vi "Destroy.vi"(8 "Error In":errorcluster, 11 "Compiler":refnum<class "Compiler.lvclass">) -> (0 "Error Out":errorcluster, 3 "Reader":refnum<class "Abstract.lvclass">)   [LabVIEW 2018, in "Toolkit.lvlib" / "Compiler.lvclass"]
uses:
  Compiler.lvclass
  Readers/Abstract/Abstract.lvclass
  Compiler.lvclass/Compiler.ctl
  Parser/Parser.lvclass
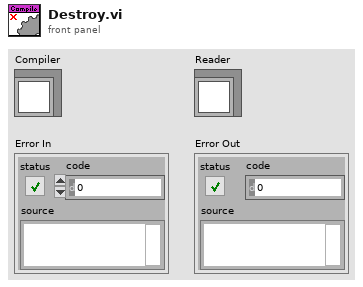
[diagram p1: front panel]
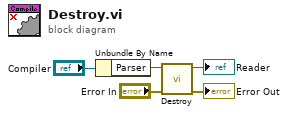
[diagram p0: block diagram]
diagram:
  n1 = Unbundle By Name("Compiler") -> ("Parser"=w4:refnum<class "Parser.lvclass">)
  n2 = call "Destroy.vi"("Error In"="Error In", "Parser"=w4) -> ("Error Out"=→"Error Out":errorcluster, "Reader"=→"Reader":refnum<class "Abstract.lvclass">)  [unwired: 8 in]
